vi "Configure Digital Output Data.vi"(5 "I Offset (0 percent)":dbl, 6 "Scaling (100 percent)":dbl=100.0, 7 "Q Offset (0 percent)":dbl, 8 "error in (no error)":errorcluster, 9 "Rotation (1 deg)":dbl=1.0, 10 "Signal Type (0: I/Q)":u16(ring) items=["I/Q", "IF"], 11 "VISA resource name":refnum<visa-resource-name>) -> (0 "error out":errorcluster, 3 "VISA resource name out":refnum<visa-resource-name>)   [LabVIEW 2012, in "Agilent PSG MXG Series.lvlib"]
doc: "Configures the N5102A output mode.\n\n<B>Notes:</B>\n(1) This VI is valid only in E8267D that installs <B>Option 601</B> or <B>Option 602</B> (Internal baseband generator), and <B>Option 003</B> (PSG digital output connectivity with N5102A).\n\n(2) This VI is valid only for the N5102A module output mode."
uses:
  <instrlib>/Agilent PSG MXG Series/Agilent PSG MXG Series.lvlib
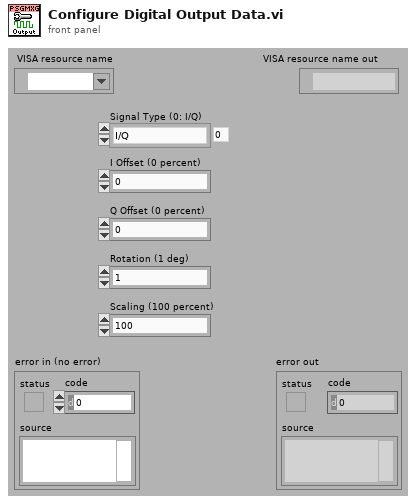
[diagram p1: front panel]
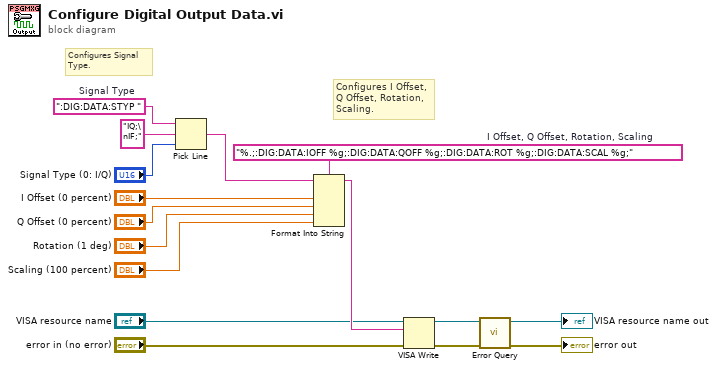
[diagram p0: block diagram]
diagram:
  w12 = "%.;:DIG:DATA:IOFF %g;:DIG:DATA:QOFF %g;:DIG:DATA:ROT %g;:DIG:DATA:SCAL %g;"  # I Offset, Q Offset, Rotation, Scaling
  w16 = ":DIG:DATA:STYP "  # Signal Type
  # "Configures I Offset,\nQ Offset, Rotation,\nScaling."
  # "Configures Signal\nType."
  n1 = Pick Line(string ("")=w16, multi-line string="IQ;\nIF;", line index="Signal Type (0: I/Q)") -> (output string=w13:string)
  n2 = Format Into String(format string=w12, initial string=w13, "I Offset (0 percent)", "Q Offset (0 percent)", "Rotation (1 deg)", "Scaling (100 percent)") -> (resulting string=w7:string)  [unwired: 1 in, 1 out]
  n3 = VISA Write(VISA resource name="VISA resource name", write buffer=w7, error in (no error)="error in (no error)") -> (VISA resource name out=w6:refnum<visa-resource-name>, error out=w5:errorcluster)  [unwired: 1 out]
  n4 = call <instrlib>:"Error Query.vi"("error in (no error)"=w5, "VISA resource name"=w6) -> ("error out"=→"error out":errorcluster, "VISA resource name out"=→"VISA resource name out":refnum<visa-resource-name>)  [unwired: 8 out]
